vi "Shutter Controls Test V1.vi"() -> ()   [LabVIEW 2014]
uses:
  <vilib>/rvi/Emulation/niFpgaGetClockAttributes.vi
  <vilib>/rvi/Emulation/niFpgaSctlEmulationGetInTimedLoop.vi
  <vilib>/rvi/Emulation/niFpgaEmulationReportErrorSimple.vi
  <vilib>/rvi/eio/common/nirviEmuTemplateMethod_errors.vi
  <vilib>/rvi/Emulation/niFpgaCriticalErrorInLSC.vi
  <vilib>/eio/EIONode/EIONode.xnode
panel:
  in  "stop":bool
  out "Upper Shutter Status":bool
  out "Lower Shutter Status":bool
  in  "Upper Shutter Command":bool
  in  "Lower Shutter Command":bool
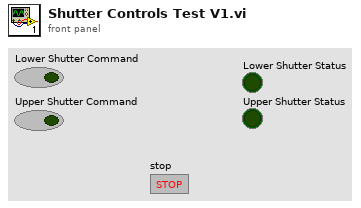
[diagram p1: front panel]
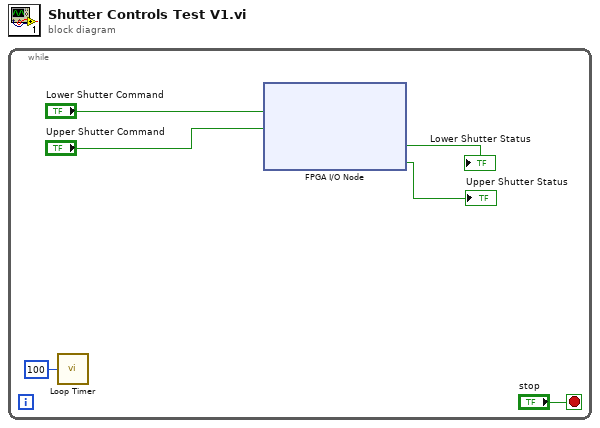
[diagram p0: block diagram]
diagram:
  n1 = while {
    stop <- "stop" stop-if-true
    n2 = call "Loop Timer"("Count(uSec)"=u32 100) -> ()  [unwired: 1 out]
    n3 = xnode "FPGA I/O Node"("Connector1/DIO26"="Lower Shutter Command", "Connector1/DIO28"="Upper Shutter Command") -> ("Connector1/DIO25"=→"Lower Shutter Status":bool, "Connector2/DIO27"=→"Upper Shutter Status":bool)  [unwired: 4 in, 4 out]
  }
